vi "Main.vi"() -> ()   [LabVIEW 2015]
doc: "This template is for the Queued Message Handler design pattern.\n\nThe Event Handling Loop generates messages based on user interface actions.\n\nThe Message Handling Loop processes messages generated by the Event Handling Loop, or by other messages. The messages are string values, so new messages can be added easily to the Message Cases case structure in the Message Handling Loop. Each message cluster can also provide an optional value for Message Data, which is a variant that can be converted to whatever message-specific data is required."
uses:
  support/Type Definitions/UI Data.ctl
  support/Status Logger/Status Log.ctl
  support/Global names.vi
  support/Message Queue/Enqueue Message (Single).vi
  <vilib>/Utility/error.llb/Error Cluster From Error Code.vi
  <vilib>/ErrorRing/Error Ring.xnode
  support/Message Queue/Message Queue.lvlib
  Support/User Event - EHL Stop/User Event - EHL Stop.lvlib
  Model/Model.lvlib
  PLC/PLC.lvlib
panel:
  out "Power status":bool
  in  "Abort":bool
  in  "Stop Line":bool
  in  "Start Line":bool
  out "Status":string
  in  "Tab Control":enum32{"Simulation"}(tab)
  in  "Power switch":bool
  in  "Positon":dbl(slide) scale=0.0..20.0
  in  "Dispose":bool
  in  "Pump":bool
  in  "Flow [l/s]":dbl=10.0
  in  "Exit":bool
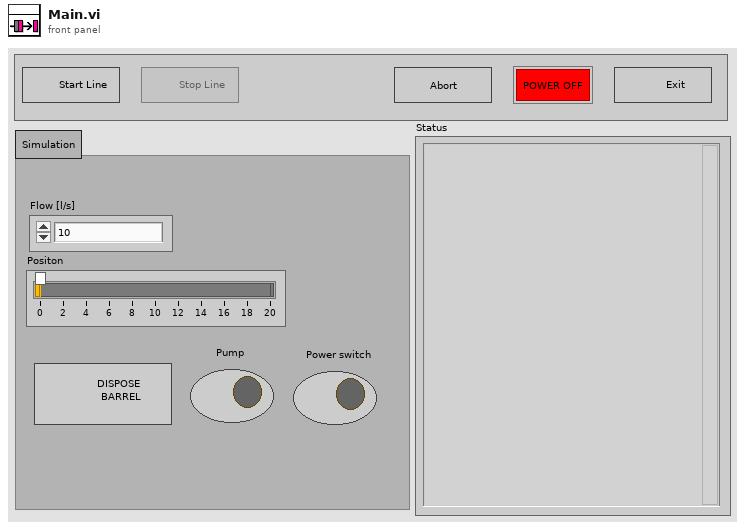
[diagram p1: front panel]
types:
  T1 = typedef "Status Log.ctl" = enum16{"Close file", "Open Status file", "Add Status", "Show Status File"}
  T2 = typedef "UI Data.ctl" = cluster{"Start Line Ref":refnum<vi>, "Stop Line Ref":refnum<vi>, "Data Display Ref":refnum<vi>, "Exit Button Ref":refnum<vi>, "Pump Ref":refnum<vi>, "Dispose Ref":refnum<vi>, "Flow Ref":refnum<vi>, "Position Ref":refnum<vi>, "Tab Ref":refnum<vi>, "Abort":refnum<vi>, "Power status":refnum<vi>, "Power switch":refnum<vi>}
  T3 = typedef "Notifiers.lvlib/Notifiers.ctl" = cluster{"PLC":refnum<notifier>, "Model":refnum<notifier>}
  T4 = typedef "Message Queue.lvlib/All Message Queues.ctl" = cluster{"UI":refnum<queue>, "Model":refnum<queue>, "PLC":refnum<queue>}
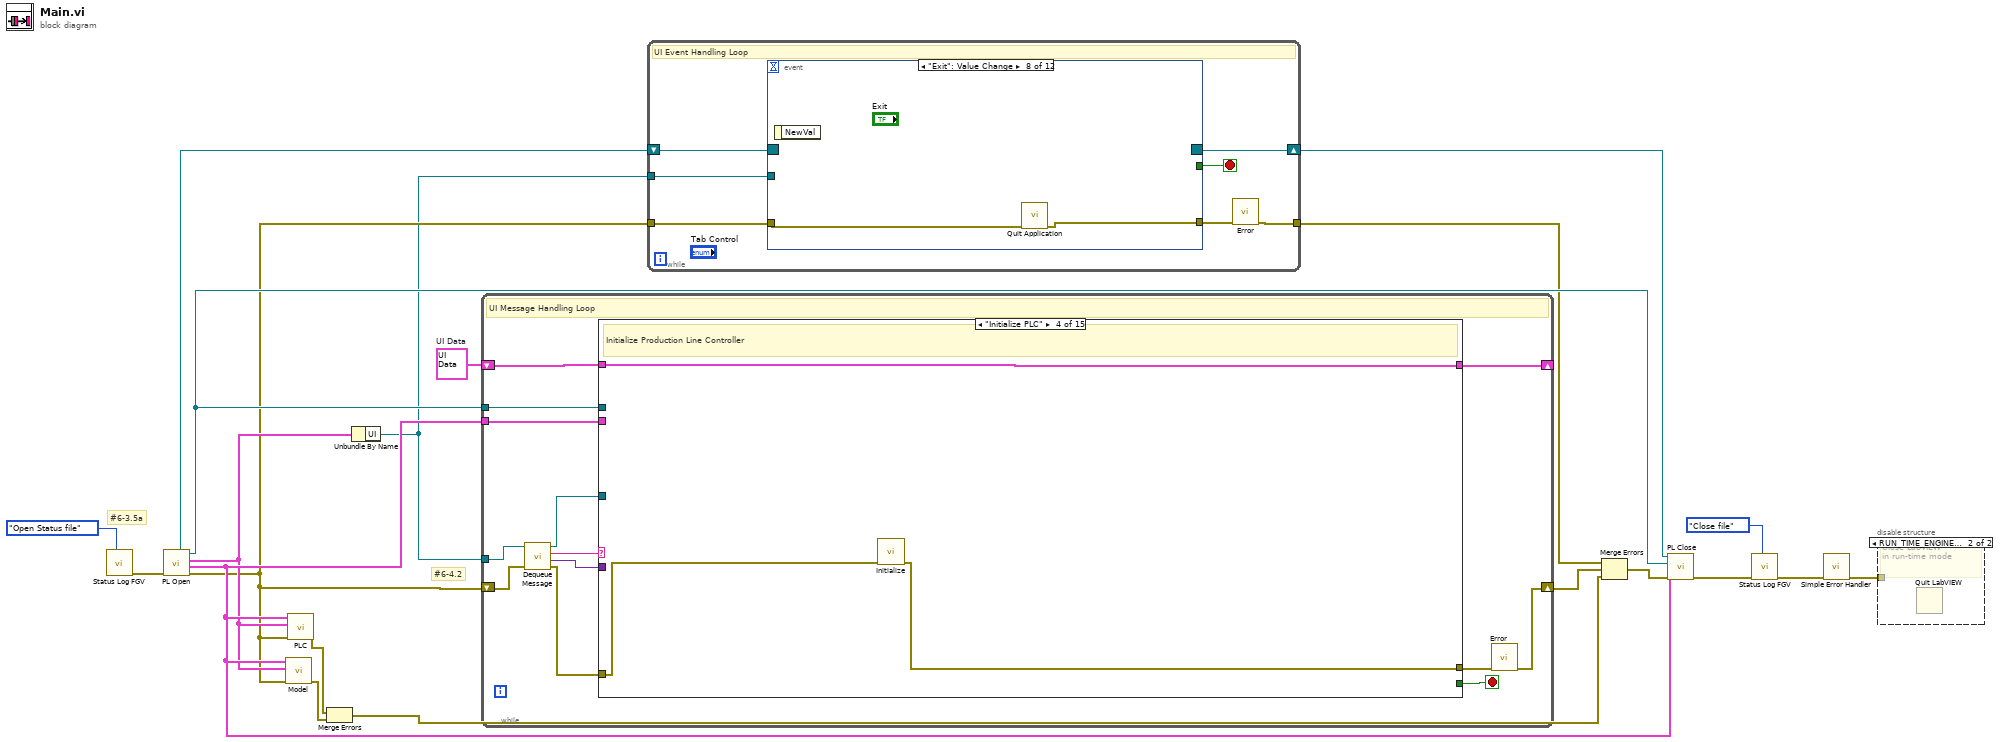
[diagram p0: block diagram]
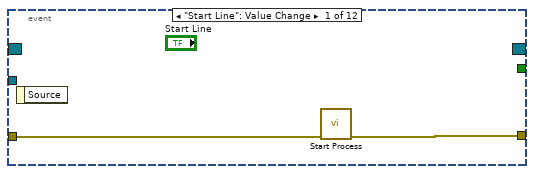
[diagram p2: hidden frame]
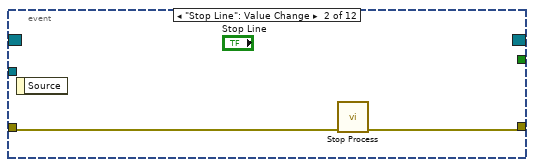
[diagram p3: hidden frame]
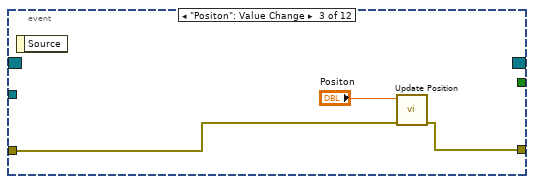
[diagram p4: hidden frame]
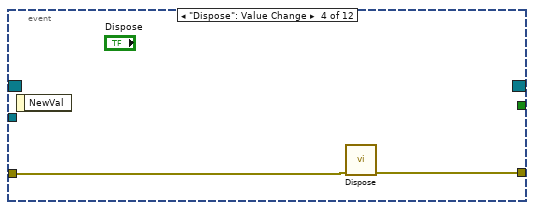
[diagram p5: hidden frame]
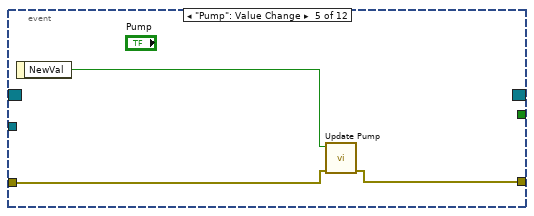
[diagram p6: hidden frame]
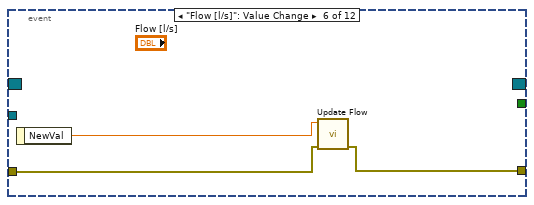
[diagram p7: hidden frame]
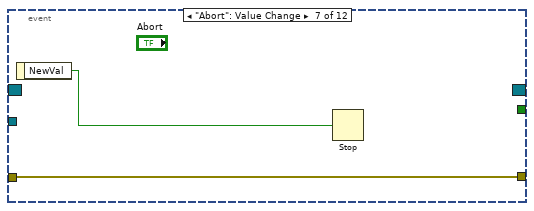
[diagram p8: hidden frame]
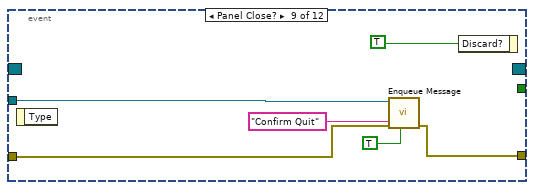
[diagram p9: hidden frame]
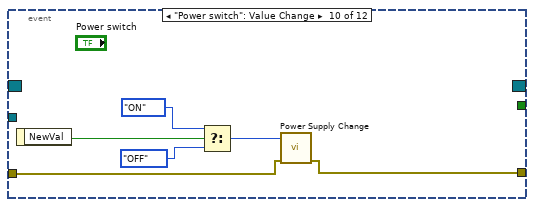
[diagram p10: hidden frame]
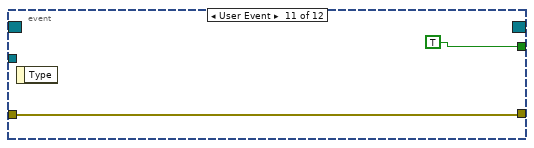
[diagram p11: hidden frame]
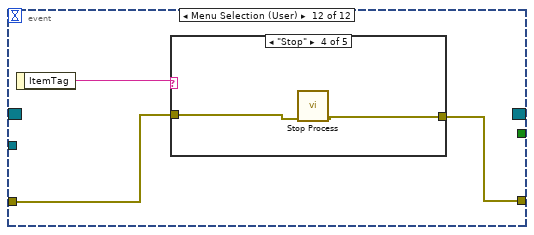
[diagram p12: hidden frame]
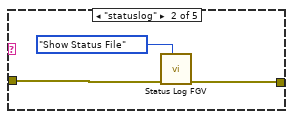
[diagram p14: hidden frame]
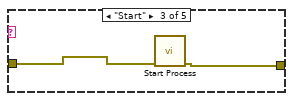
[diagram p15: hidden frame]
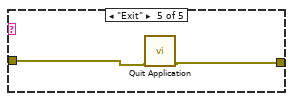
[diagram p16: hidden frame]
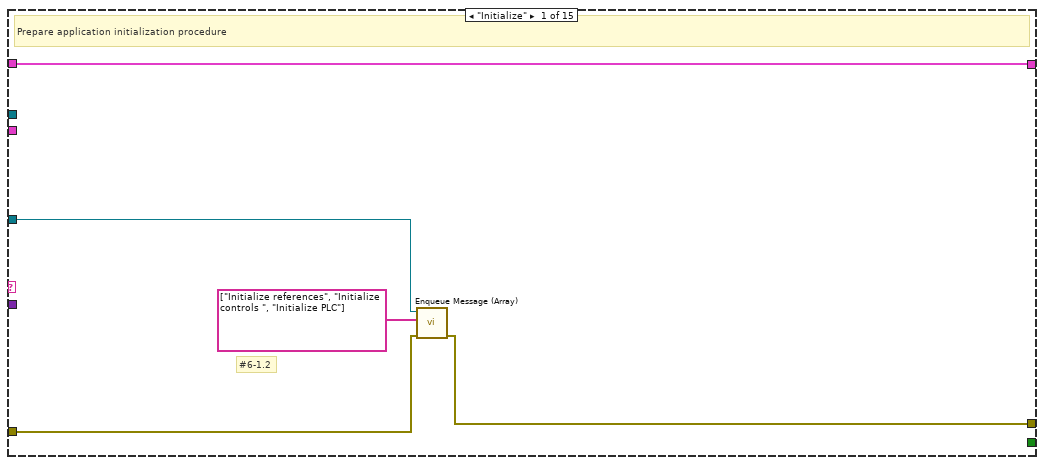
[diagram p18: hidden frame]
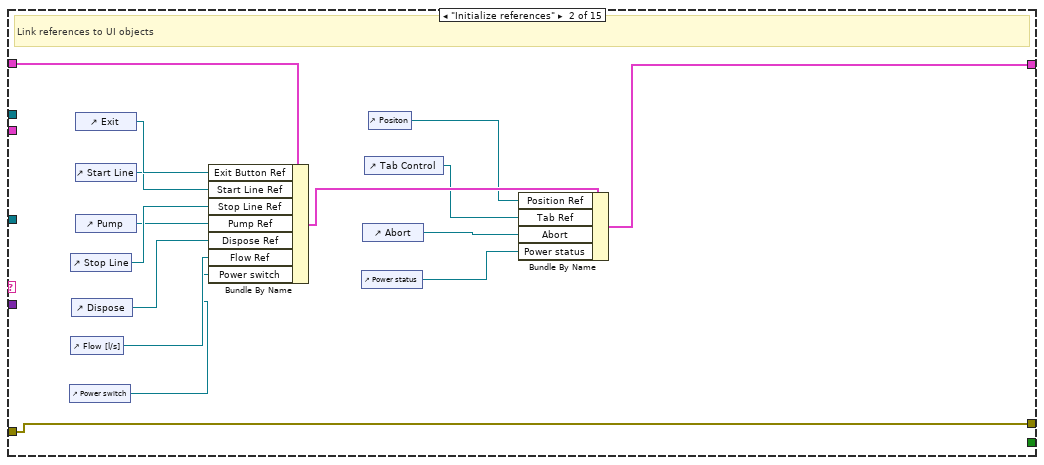
[diagram p19: hidden frame]
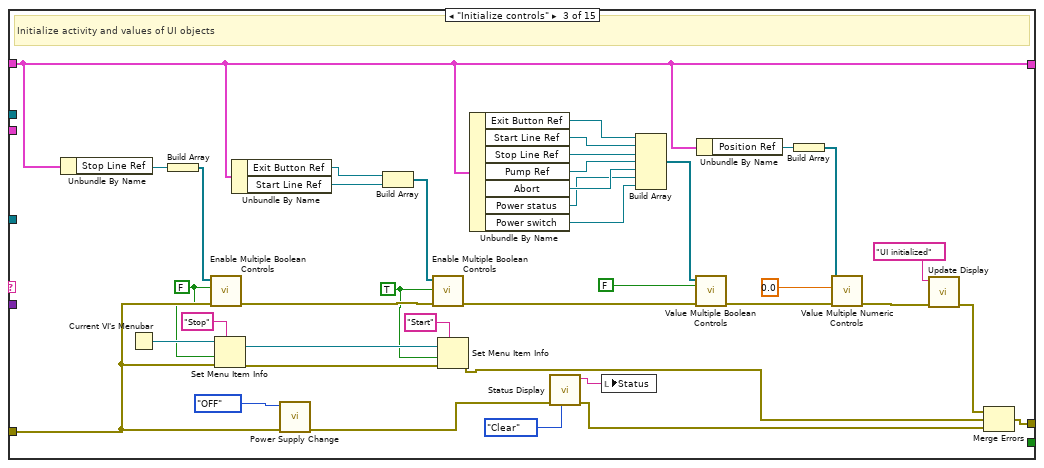
[diagram p20: hidden frame]
diagram:
  w19 = T2 {"Start Line Ref"=refnum, "Stop Line Ref"=refnum, "Data Display Ref"=refnum, "Exit Button Ref"=refnum, "Pump Ref"=refnum, "Dispose Ref"=refnum, "Flow Ref"=refnum, "Position Ref"=refnum, "Tab Ref"=refnum, "Abort"=refnum, "Power status"=refnum, "Power switch"=refnum}  # UI Data
  # "#6-3.5a"
  # "#6-4.2"
  n1 = call "Status Log FGV.vi"("Action"=Status_Log."Open Status file") -> ("error out"=w2:errorcluster)  [unwired: 10 in]
  n2 = call "PL Open.vi"("error in"=w2) -> ("error out"=w4:errorcluster, "Notifiers"=w9:T3, "Queues"=w8:T4, "User Event"=w17:refnum<user-event>, "Event Registration Refnum"=w11:refnum<event-registration>)  [unwired: 6 in]
  n3 = call "Model.vi"("error in"=w4, "Queues"=w8, "Notifiers"=w9) -> ("error out"=w6:errorcluster)  [unwired: 8 in]
  n4 = call "PLC.vi"("error in"=w4, "Message Queues"=w8, "Notifiers"=w9) -> ("error out"=w7:errorcluster)  [unwired: 8 in]
  n5 = Merge Errors(w7, w6) -> (w5:errorcluster)
  n6 = Unbundle By Name(w8) -> ("UI"=w3:refnum<queue>)
  n7 = while {
    shift-right: [w32] -> _
    shift-left: w19 -> [w33]
    tunnel: w17 -> [w30]
    tunnel: w9 -> [w26]
    shift-right: [w22] -> w15
    shift-left: w4 -> [w29]
    tunnel: w3 -> [w24]
    stop <- w31 stop-if-true
    # "UI Message Handling Loop"
    n8 = call "Dequeue Message.vi"("error in (no error)"=w29, "Message Queue"=w24) -> ("error out"=w28:errorcluster, "Message Data"=w25:variant, "Message"=w21:string, "dup Message Queue"=w27:refnum<queue>)  [unwired: 6 in]
    n9 = case "Message Cases" shown="\"Initialize PLC\"" w21 {
      selector: w21 -> [_ _ _ _ _ _ _ _ _ _ _ _ _ _ w249]
      tunnel: w27 -> [w36 _ _ _ _ _ _ _ _ _ w195 w201 w237 _ _]
      tunnel: w28 -> [w37 w42 w62 w93 w109 w127 w141 w157 w185 w187 w196 w203 w220 w244 _]
      tunnel: [w35 w42 w71 w94 w108 w129 w145 w158 w179 w186 w193 w200 w224 w238 w248] -> w23
      tunnel: w33 -> [w38 w53 w79 w95 w114 w139 w149 w161 w182 w191 w197 w207 w229 w243 w250]
      tunnel: [w38 w43 w79 w95 w114 w139 w149 w161 w182 w191 w197 w207 w229 w243 w250] -> w32
      tunnel: [_ _ _ _ _ _ _ _ _ _ _ _ TRUE _ _] -> w31
      tunnel: w25 -> [_ _ _ _ _ _ w152 w155 w184 w190 _ _ w231 _ _]
      tunnel: w30 -> [_ _ _ _ _ _ _ _ _ _ _ _ w234 _ _]
      tunnel: w26 -> [_ _ _ _ _ _ _ _ _ _ _ w206 _ _ _]
      frame "Initialize" {
        # "#6-1.2"
        # "Prepare application initialization procedure"
        n10 = call "Enqueue Message (Array).vi"("error in (no error)"=w37, "Message Array"=string[] ["Initialize references", "Initialize controls ", "Initialize PLC"], "Message Queue"=w36) -> ("error out"=w35:errorcluster)  [unwired: 7 in, 1 out]
      }
      frame "Initialize references" {
        # "Link references to UI objects"
        n11 = control-ref of="Power switch"() -> (w41:refnum<vi>)
        n12 = control-ref of="Stop Line"() -> (w50:refnum<vi>)
        n13 = control-ref of="Flow [l/s]"() -> (w47:refnum<vi>)
        n14 = control-ref of="Dispose"() -> (w48:refnum<vi>)
        n15 = control-ref of="Exit"() -> (w52:refnum<vi>)
        n16 = control-ref of="Start Line"() -> (w51:refnum<vi>)
        n17 = control-ref of="Pump"() -> (w49:refnum<vi>)
        n18 = Bundle By Name(cluster=w53, "Exit Button Ref"=w52, "Start Line Ref"=w51, "Stop Line Ref"=w50, "Pump Ref"=w49, "Dispose Ref"=w48, "Flow Ref"=w47, "Power switch"=w41) -> (w46:T2)
        n19 = control-ref of="Power status"() -> (w39:refnum<vi>)
        n20 = control-ref of="Abort"() -> (w40:refnum<vi>)
        n21 = control-ref of="Tab Control"() -> (w44:refnum<vi>)
        n22 = control-ref of="Positon"() -> (w45:refnum<vi>)
        n23 = Bundle By Name(cluster=w46, "Position Ref"=w45, "Tab Ref"=w44, "Abort"=w40, "Power status"=w39) -> (w43:T2)
      }
      frame "Initialize controls" {
        w54 = TRUE ("Enabled")
        w55 = FALSE ("Enabled")
        # "Initialize activity and values of UI objects"
        n24 = Unbundle By Name(w79) -> ("Stop Line Ref"=w92:refnum<vi>)
        n25 = Current VI's Menubar() -> (w57:refnum<k9>)
        n26 = Build Array(w92) -> (w91:refnum<vi>[])
        n27 = call "Enable Multiple Boolean Controls.vi"("error in"=w62, "Enabled"=w55, "References"=w91) -> ("error out"=w88:errorcluster)  [unwired: 8 in]
        n28 = Set Menu Item Info(7:"Stop" ("item tag"), 8:w62, 9:w55, 11:w57) -> (0:w60:errorcluster, 3:w56:refnum<k9>)  [unwired: 3 in]
        n29 = Unbundle By Name(w79) -> ("Exit Button Ref"=w90:refnum<vi>, "Start Line Ref"=w89:refnum<vi>)
        n30 = call "Power Supply Change.vi"("error in"=w62, "Power status"=enum16{"OFF", "ON"}."OFF") -> ("error out"=w68:errorcluster)  [unwired: 9 in]
        n31 = Build Array(w90, w89) -> (w87:refnum<vi>[])
        n32 = call "Enable Multiple Boolean Controls.vi"("error in"=w88, "Enabled"=w54, "References"=w87) -> ("error out"=w82:errorcluster)  [unwired: 8 in]
        n33 = Set Menu Item Info(7:"Start" ("item tag"), 8:w60, 9:w54, 11:w56) -> (0:w58:errorcluster)  [unwired: 3 in, 1 out]
        n34 = Unbundle By Name(w79) -> ("Exit Button Ref"=w86:refnum<vi>, "Start Line Ref"=w85:refnum<vi>, "Stop Line Ref"=w84:refnum<vi>, "Pump Ref"=w83:refnum<vi>, "Abort"=w74:refnum<vi>, "Power status"=w73:refnum<vi>, "Power switch"=w64:refnum<vi>)
        n35 = call "Status Display.vi"("Action"=enum16{"Update", "Clear"}."Clear", "error in"=w68) -> ("error out"=w67:errorcluster, "Status"=w65:string)  [unwired: 8 in]
        n36 = local write "Status"(w65) -> ()
        n37 = Build Array(w86, w85, w84, w83, w74, w73, w64) -> (w80:refnum<vi>[])
        n38 = call "Value Multiple Boolean Controls.vi"("error in"=w82, "Value"=FALSE ("Enabled"), "References"=w80) -> ("error out"=w78:errorcluster)  [unwired: 8 in]
        n39 = Unbundle By Name(w79) -> ("Position Ref"=w77:refnum<vi>)
        n40 = Build Array(w77) -> (w76:refnum<vi>[])
        n41 = call "Value Multiple Numeric Controls.vi"("error in"=w78, "Value"=0.0, "References"=w76) -> ("error out"=w70:errorcluster)  [unwired: 8 in]
        n42 = call "Update Display.vi"("error in"=w70, "Message string"="UI initialized") -> ("error out"=w59:errorcluster)  [unwired: 9 in]
        n43 = Merge Errors(w59, w58, w67) -> (w71:errorcluster)
      }
      frame "Initialize PLC" {
        # "Initialize Production Line Controller"
        n44 = call "Initialize.vi"("error in"=w93) -> ("error out"=w94:errorcluster)  [unwired: 10 in]
      }
      frame "Start process" {
        w100 = TRUE ("Enabled")
        w104 = FALSE ("Enabled")
        # "Starts process: start PLC, open logger file, create reports files, enable/disable UI controls and update status display"
        n45 = Unbundle By Name(w114) -> ("Exit Button Ref"=w97:refnum<vi>, "Start Line Ref"=w110:refnum<vi>, "Stop Line Ref"=w113:refnum<vi>)
        n46 = Build Array(w97, w110) -> (w115:refnum<vi>[])
        n47 = Build Array(w113) -> (w112:refnum<vi>[])
        n48 = call "Start.vi"("error in"=w109) -> ("error out"=w111:errorcluster)  [unwired: 10 in]
        n49 = call "Enable Multiple Boolean Controls.vi"("error in"=w109, "Enabled"=w100, "References"=w112) -> ("error out"=w102:errorcluster)  [unwired: 8 in]
        n50 = call "Enable Multiple Boolean Controls.vi"("error in"=w109, "Enabled"=w104, "References"=w115) -> ("error out"=w106:errorcluster)  [unwired: 8 in]
        n51 = global read "Global names.vi" "Starting"() -> (w98:string)
        n52 = Current VI's Menubar() -> (w99:refnum<k9>)
        n53 = call "Update Display.vi"("error in"=w111, "Message string"=w98) -> ("error out"=w96:errorcluster)  [unwired: 9 in]
        n54 = Set Menu Item Info(7:"Start" ("item tag"), 8:w106, 9:w104, 11:w99) -> (0:w105:errorcluster)  [unwired: 3 in, 1 out]
        n55 = Set Menu Item Info(7:"Stop" ("item tag"), 8:w102, 9:w100, 11:w99) -> (0:w101:errorcluster)  [unwired: 3 in, 1 out]
        n56 = Merge Errors(w96, w105, w101) -> (w108:errorcluster)
      }
      frame "Stop process" {
        w118 = FALSE ("Enabled")
        w119 = TRUE ("Enabled")
        # "Stops process: stop PLC, close logger file, save and close report files, enable/disable UI controls and update status display"
        n57 = Unbundle By Name(w139) -> ("Exit Button Ref"=w116:refnum<vi>, "Start Line Ref"=w132:refnum<vi>, "Stop Line Ref"=w138:refnum<vi>)
        n58 = call "Stop.vi"("error in"=w127) -> ("error out"=w134:errorcluster)  [unwired: 10 in]
        n59 = Build Array(w138) -> (w128:refnum<vi>[])
        n60 = Build Array(w116, w132) -> (w136:refnum<vi>[])
        n61 = global read "Global names.vi" "Stopping"() -> (w117:string)
        n62 = Build Array (concatenate)(w136, w128) -> (w135:refnum<vi>[])
        n63 = call "Enable Multiple Boolean Controls.vi"("error in"=w127, "Enabled"=w119, "References"=w136) -> ("error out"=w124:errorcluster)  [unwired: 8 in]
        n64 = call "Enable Multiple Boolean Controls.vi"("error in"=w127, "Enabled"=w118, "References"=w128) -> ("error out"=w131:errorcluster)  [unwired: 8 in]
        n65 = call "Value Multiple Boolean Controls.vi"("error in"=w127, "Value"=FALSE, "References"=w135) -> ("error out"=w130:errorcluster)  [unwired: 8 in]
        n66 = call "Update Display.vi"("error in"=w134, "Message string"=w117) -> ("error out"=w133:errorcluster)  [unwired: 9 in]
        n67 = Current VI's Menubar() -> (w125:refnum<k9>)
        n68 = Set Menu Item Info(7:"Start" ("item tag"), 8:w124, 9:w119, 11:w125) -> (0:w122:errorcluster, 3:w120:refnum<k9>)  [unwired: 3 in]
        n69 = Set Menu Item Info(7:"Stop" ("item tag"), 8:w122, 9:w118, 11:w120) -> (0:w121:errorcluster)  [unwired: 3 in, 1 out]
        n70 = Merge Errors(w133, w121, w131, w130) -> (w129:errorcluster)
      }
      frame "Update display" {
        # "#6-3.5b"
        # "Updates status display, status log file and word report file"
        n71 = Variant To Data(error in=w141, type="", Variant=w152) -> (data=w143:string, error out=w144:errorcluster)
        n72 = call "Status Log FGV.vi"("Action"=Status_Log."Add Status", "error in"=w144, "Status"=w143) -> ("error out"=w140:errorcluster)  [unwired: 8 in]
        n73 = call "Status Display.vi"("Action"=enum16{"Update", "Clear"}."Update", "error in"=w144, "Status line"=w143) -> ("error out"=w146:errorcluster, "Status"=→"Status":string)  [unwired: 7 in]
        n74 = property on="Status" class="Str"("Text.Scroll Position"=-1) -> ()  [unwired: 2 in, 2 out]
        n75 = Merge Errors(w141, w140, w146) -> (w145:errorcluster)
      }
      frame "Update position" {
        # "Programmatically update position of the barrel slider"
        n76 = Variant To Data(error in=w157, type=0.0 ("Value"), Variant=w155) -> (data=w153:dbl, error out=w156:errorcluster)
        n77 = Unbundle By Name(w161) -> ("Position Ref"=w160:refnum<vi>)
        n78 = Build Array(w160) -> (w159:refnum<vi>[])
        n79 = call "Value Multiple Numeric Controls.vi"("error in"=w156, "Value"=w153, "References"=w159) -> ("error out"=w158:errorcluster)  [unwired: 8 in]
      }
      frame "Power status change" {
        # "Update main switch LED and Start/Stop buttons according to power status change (DAQ DI)"
        n80 = Variant To Data(error in=w185, type=TRUE, Variant=w184) -> (data=w162:bool, error out=w166:errorcluster)
        "Power status" <- w162
        n81 = Unbundle By Name(w182) -> ("Start Line Ref"=w181:refnum<vi>, "Stop Line Ref"=w180:refnum<vi>)
        n82 = Build Array(w181) -> (w178:refnum<vi>[])
        n83 = Build Array(w180) -> (w175:refnum<vi>[])
        n84 = Build Array (concatenate)(w178, w175) -> (w177:refnum<vi>[])
        n85 = Current VI's Menubar() -> (w169:refnum<k9>)
        n86 = call "Enable Multiple Boolean Controls.vi"("error in"=w166, "Enabled"=w162, "References"=w178) -> ("error out"=w173:errorcluster)  [unwired: 8 in]
        n87 = Set Menu Item Info(7:"Start" ("item tag"), 8:w166, 9:w162, 11:w169) -> (0:w167:errorcluster, 3:w163:refnum<k9>)  [unwired: 3 in]
        n88 = call "Value Multiple Boolean Controls.vi"("error in"=w166, "Value"=FALSE, "References"=w177) -> ("error out"=w172:errorcluster)  [unwired: 8 in]
        n89 = call "Enable Multiple Boolean Controls.vi"("error in"=w166, "Enabled"=FALSE, "References"=w175) -> ("error out"=w171:errorcluster)  [unwired: 8 in]
        n90 = Set Menu Item Info(7:"Stop" ("item tag"), 8:w167, 9:FALSE ("enabled"), 11:w163) -> (0:w164:errorcluster)  [unwired: 3 in, 1 out]
        n91 = Merge Errors(w173, w172, w171, w164) -> (w179:errorcluster)
      }
      frame "Error" {
        # "Display error dialog box and quit application"
        n92 = Variant To Data(error in=w187, type=errorcluster {"status"=FALSE, "code"=0, "source"=""} ("error constant"), Variant=w190) -> (data=w188:errorcluster, error out=w186:errorcluster)
        n93 = call <vilib>:"Simple Error Handler.vi"("error in (no error)"=w188) -> ()  [unwired: 4 in, 5 out]
      }
      frame "Exit" {
        # "Start exit procedure: stop PLC, then send Exit message to PLC and go to PLC confirmation loop"
        n94 = Flush Queue(queue=w195, error in (no error)=w196) -> (error out=w192:errorcluster)  [unwired: 2 out]
        n95 = call "Exit PLC.vi"("error in"=w192) -> ("error out"=w194:errorcluster)  [unwired: 10 in]
        n96 = call "Wait on PLC Exit.vi"("error in"=w194) -> ("error out"=w193:errorcluster)  [unwired: 10 in]
      }
      frame "Wait on PLC exit" {
        # "Wait until PLC shutdown"
        n97 = Unbundle By Name(w206) -> ("PLC"=w205:refnum<notifier>)
        n98 = Wait on Notification(notifier=w205, timeout in ms (-1)=10, error in (no error)=w203) -> (notification=w199:string, timed out?=w202:bool, error out=w198:errorcluster)  [unwired: 1 in, 1 out]
        n99 = case shown="True" w202 {
          tunnel: [w208 w217] -> w200
          tunnel: w198 -> [w209 w214]
          tunnel: w201 -> [_ w215]
          tunnel: w199 -> [_ w210]
          frame True {
            # "Shutdown notification from PLC not received"
            n100 = call "Wait on PLC Exit.vi"("error in"=w209) -> ("error out"=w208:errorcluster)  [unwired: 10 in]
          }
          frame False {
            # "Shutdown notification from PLC received (handshake)"
            n101 = call "Update Display.vi"("error in"=w214, "Message string"=w210) -> ("error out"=w213:errorcluster)  [unwired: 9 in]
            n102 = call "Update Display.vi"("error in"=w213, "Message string"="Application quits" ("Message")) -> ("error out"=w212:errorcluster)  [unwired: 9 in]
            n103 = call-poly "Enqueue Message.vi"("error in (no error)"=w212, "Message"="End program", "Message Queue"=w215) -> ("error out"=w217:errorcluster)  [unwired: 7 in, 1 out]
          }
        }
      }
      frame "End program" {
        # "Shutdown MHL and send exit user event to EHL; reset UI controls"
        n104 = call "Fire User Event - EHL Stop.vi"("error in (no error)"=w220, "User Event - Stop"=w234) -> ("error out"=w219:errorcluster)  [unwired: 9 in]
        n105 = Variant To Data(error in=w220, type=errorcluster {"status"=FALSE, "code"=0, "source"=""} ("error constant"), Variant=w231) -> (data=w232:errorcluster)  [unwired: 1 out]
        n106 = Release Queue(queue=w237, force destroy? (F)=TRUE, error in (no error)=w220) -> (error out=w235:errorcluster)  [unwired: 2 out]
        n107 = call <vilib>:"Simple Error Handler.vi"("error in (no error)"=w232) -> ("error out"=w218:errorcluster)  [unwired: 4 in, 4 out]
        n108 = Merge Errors(w219, w218, w235) -> (w225:errorcluster)
        n109 = Unbundle By Name(w229) -> ("Exit Button Ref"=w228:refnum<vi>, "Abort"=w223:refnum<vi>, "Start Line Ref"=w222:refnum<vi>, "Stop Line Ref"=w221:refnum<vi>)
        n110 = Build Array(w228, w223, w222, w221) -> (w227:refnum<vi>[])
        n111 = call "Value Multiple Boolean Controls.vi"("error in"=w225, "Value"=FALSE, "References"=w227) -> ("error out"=w224:errorcluster)  [unwired: 8 in]
      }
      frame "Confirm Quit" {
        # "Confirm Quit - Message that can confirm whether or not the user wants to exit the application."
        n112 = Two Button Dialog(message="Are you sure?", 1:"Continue" ("F button name (\"Cancel\")"), 2:"Quit" ("T button name (\"OK\")")) -> (T button?=w239:bool)
        n113 = case shown="True" w239 {
          tunnel: w244 -> [w245 w247]
          tunnel: [w245 w246] -> w238
          frame False {
          }
          frame True {
            n114 = call "Quit Application.vi"("error in"=w247) -> ("error out"=w246:errorcluster)  [unwired: 10 in]
          }
        }
      }
      frame Default {
        # "Incorrect message: show error and clear error"
        n115 = xnode "Error Ring"("parameter 0"=w249) -> ("error out"=w248:errorcluster)
      }
    }
    n116 = call "Error.vi"("error in"=w23) -> ("error out"=w22:errorcluster)  [unwired: 10 in]
  }
  n117 = while {
    tunnel: w3 -> [w260]
    shift-right: [w263] -> w20
    shift-left: w11 -> [w264]
    tunnel: [w258] -> w10
    tunnel: w4 -> [w261]
    stop <- w262 stop-if-true
    # "UI Event Handling Loop"
    n118 = event shown="[7] \"Exit\": Value Change" {
      selector: w264 -> [_ _ _ _ _ _ _ _ _ _ _ _]
      dyn-events: [_ _ _ _ _ _ _ _ _ _ _ _] -> w263
      timeout: _ -> [_ _ _ _ _ _ _ _ _ _ _ _]
      tunnel: [_ _ _ _ _ _ _ _ _ _ TRUE ("Discard?") _] -> w262
      tunnel: w260 -> [_ _ _ _ _ _ _ _ w289 _ _ _]
      tunnel: [w265 w267 w270 w272 w275 w278 w281 w282 w288 w290 w296 w299] -> w259
      tunnel: w261 -> [w266 w268 w269 w273 w276 w279 w281 w283 w284 w291 w296 w298]
      event "Start Line": Value Change {
        n119 = event-data() -> ()  [unwired: 1 in, 1 out]
        n120 = call "Start Process.vi"("error in"=w266) -> ("error out"=w265:errorcluster)  [unwired: 10 in]
      }
      event "Stop Line": Value Change {
        n121 = event-data() -> ()  [unwired: 1 in, 1 out]
        n122 = call "Stop Process.vi"("error in"=w268) -> ("error out"=w267:errorcluster)  [unwired: 10 in]
      }
      event "Positon": Value Change {
        n123 = event-data() -> ()  [unwired: 1 in, 1 out]
        n124 = call "Update Position.vi"("error in (no error)"=w269, "Position"="Positon") -> ("error out"=w270:errorcluster)  [unwired: 9 in]
      }
      event "Dispose": Value Change {
        n125 = event-data() -> ()  [unwired: 1 in, 1 out]
        n126 = call "Dispose.vi"("error in (no error)"=w273) -> ("error out"=w272:errorcluster)  [unwired: 10 in]
      }
      event "Pump": Value Change {
        n127 = event-data() -> ("NewVal"=w274:bool)  [unwired: 1 in]
        n128 = call "Update Pump.vi"("error in (no error)"=w276, "Pump State"=w274) -> ("error out"=w275:errorcluster)  [unwired: 9 in]
      }
      event "Flow [l/s]": Value Change {
        n129 = event-data() -> ("NewVal"=w277:dbl)  [unwired: 1 in]
        n130 = call "Update Flow.vi"("error in (no error)"=w279, "Flow"=w277) -> ("error out"=w278:errorcluster)  [unwired: 9 in]
      }
      event "Abort": Value Change {
        n131 = event-data() -> ("NewVal"=w280:bool)  [unwired: 1 in]
        n132 = Stop(stop? (T)=w280) -> ()
      }
      event "Exit": Value Change {
        n133 = event-data() -> ()  [unwired: 1 in, 1 out]
        n134 = call "Quit Application.vi"("error in"=w283) -> ("error out"=w282:errorcluster)  [unwired: 10 in]
      }
      event Panel Close? {
        n135 = event-data() -> ()  [unwired: 1 in, 1 out]
        n136 = call-poly "Enqueue Message.vi"("Priority Message? (F)"=TRUE, "error in (no error)"=w284, "Message"="Confirm Quit", "Message Queue"=w289) -> ("error out"=w288:errorcluster)  [unwired: 6 in, 1 out]
        n137 = event-data("Discard?"=TRUE) -> ()  [unwired: 1 in, 1 out]
      }
      event "Power switch": Value Change {
        n138 = event-data() -> ("NewVal"=w295:bool)  [unwired: 1 in]
        n139 = Select(t=enum16{"OFF", "ON"}."ON" ("Power status"), s=w295, f=enum16{"OFF", "ON"}."OFF" ("Power status")) -> (s? t:f=w292:enum16{"OFF", "ON"})
        n140 = call "Power Supply Change.vi"("error in"=w291, "Power status"=w292) -> ("error out"=w290:errorcluster)  [unwired: 9 in]
      }
      event User Event {
        n141 = event-data() -> ()  [unwired: 1 in, 1 out]
      }
      event Menu Selection (User) {
        n142 = event-data() -> ("ItemTag"=w300:string)  [unwired: 1 in]
        n143 = case shown="\"Stop\"" w300 {
          tunnel: [w301 w302 w306 w307 w309] -> w299
          tunnel: w298 -> [w301 w303 w305 w308 w310]
          frame Default {
          }
          frame "statuslog" {
            n144 = call "Status Log FGV.vi"("Action"=Status_Log."Show Status File", "error in"=w303) -> ("error out"=w302:errorcluster)  [unwired: 9 in]
          }
          frame "Start" {
            n145 = call "Start Process.vi"("error in"=w305) -> ("error out"=w306:errorcluster)  [unwired: 10 in]
          }
          frame "Stop" {
            n146 = call "Stop Process.vi"("error in"=w308) -> ("error out"=w307:errorcluster)  [unwired: 10 in]
          }
          frame "Exit" {
            n147 = call "Quit Application.vi"("error in"=w310) -> ("error out"=w309:errorcluster)  [unwired: 10 in]
          }
        }
      }
    }
    n148 = call "Error.vi"("error in"=w259) -> ("error out"=w258:errorcluster)  [unwired: 10 in]
  }
  n149 = Merge Errors(w10, w15, w5) -> (w14:errorcluster)
  n150 = call "PL Close.vi"("error in"=w14, "Notifiers"=w9, "User Event"=w17, "Event Registration Refnum in"=w20) -> ("error out"=w18:errorcluster)  [unwired: 7 in]
  n151 = call "Status Log FGV.vi"("Action"=Status_Log."Close file", "error in"=w18) -> ("error out"=w12:errorcluster)  [unwired: 9 in]
  n152 = call <vilib>:"Simple Error Handler.vi"("error in (no error)"=w12) -> ("error out"=w13:errorcluster)  [unwired: 4 in, 4 out]
  n153 = disable-structure shown="RUN_TIME_ENGINE==True" {
    disable-tunnel: w13 -> [_ _]
    frame condition #0 (active) {
    }
    frame condition #1 {
      # "Close LabVIEW\nin run-time mode"
      n154 = Quit LabVIEW() -> ()  [unwired: 1 in]
    }
  }
